vi "Read Raw Data.vi"(8 "error in (no error)":errorcluster, 11 "1553 Board in":refnum<class "1553 Session.lvclass">) -> (0 "error out":errorcluster, 1 "Raw Data":u64[][](array[numeric]), 2 "Parameters":string[][](array[string]), 3 "1553 Board out":refnum<class "1553 Session.lvclass">)   [LabVIEW 2020, in "BCI-1553 API.lvlib" / "1553 Session.lvclass"]
doc: "Reads all the configured parameters for a 1553 Session. Each row is a unique component, while each column is a unique parameter that has been assigned to a Component in the 1553 Session.\n\nThis read will return the raw values stored for each parameter as a U64 value. It is advised to use the scaled read instead of this method."
uses:
  1553 Session.lvclass
  1553 Session.lvclass/1553 Session.ctl
  1553 Component/1553 Component.lvclass
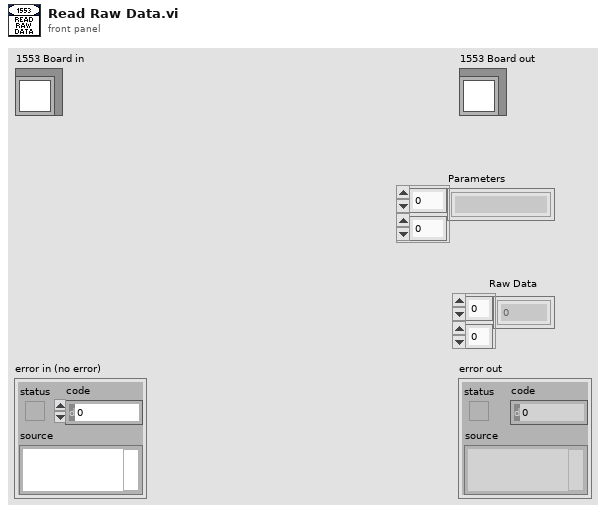
[diagram p1: front panel]
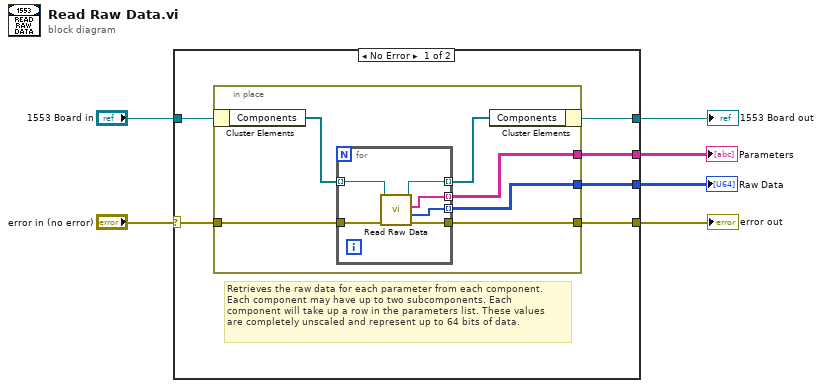
[diagram p0: block diagram]
diagram:
  n1 = case shown="No Error" "error in (no error)" {
    selector: "error in (no error)" -> [w10 w26]
    tunnel: [w9 w26] -> w5
    tunnel: [w7 w25] -> w3
    tunnel: "1553 Board in" -> [w8 w25]
    tunnel: [w12 _] -> w2
    tunnel: [w11 _] -> w1
    frame No Error {
      # "Retrieves the raw data for each parameter from each component.\nEach component may have up to two subcomponents. Each\ncomponent will take up a row in the parameters list. These values\nare completely unscaled and represent up to 64 bits of data."
      n2 = in-place {
        in-place-border: [w18] -> w12
        in-place-border: [w17] -> w11
        in-place-border: w10 -> [w16]
        in-place-border: [w15] -> w9
        n3 = in-place-cluster #1(w8) -> ("Components"=w14:refnum<class "1553 Component.lvclass">[])
        n4 = for {
          tunnel: w14 -> [w24] mode=indexing
          tunnel: w16 -> [w23]
          tunnel: [w22] -> w13 mode=indexing
          tunnel: [w21] -> w15
          tunnel: [w20] -> w18 mode=indexing
          tunnel: [w19] -> w17 mode=indexing
          n5 = call-dynamic "Read Raw Data.vi"("error in (no error)"=w23, "1553 Component in"=w24) -> ("error out"=w21:errorcluster, "Raw Data"=w19:u64[], "Parameters"=w20:string[], "1553 Component out"=w22:refnum<class "1553 Component.lvclass">)  [unwired: 6 in]
        }
        n6 = in-place-cluster #1("Components"=w13) -> (w7:refnum<class "1553 Session.lvclass">)
      }
    }
    frame Error {
    }
  }
  "error out" <- w5
  "1553 Board out" <- w3
  "Raw Data" <- w1
  "Parameters" <- w2
